vi "Configure Voltage Output.vi"(7 "Triggered Voltage (0 V)":dbl, 8 "error in (no error)":errorcluster, 9 "Immediate Voltage (0 V)":dbl, 10 "Transient Mode (0: Fixed)":i32(ring) items=["Fixed", "Step"], 11 "VISA resource name":refnum<visa-resource-name>) -> (0 "error out":errorcluster, 3 "VISA resource name out":refnum<visa-resource-name>)   [LabVIEW 2017, in "Keysight N8900 Series.lvlib"]
doc: "Configures the voltage transient mode and output voltage level."
uses:
  Keysight N8900 Series.lvlib
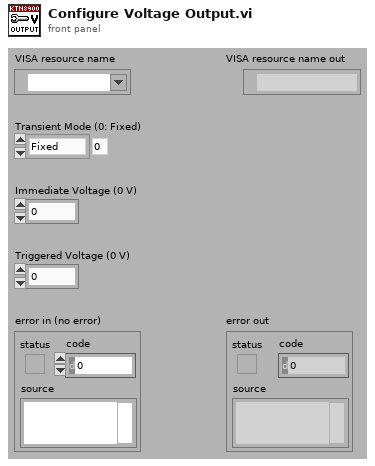
[diagram p1: front panel]
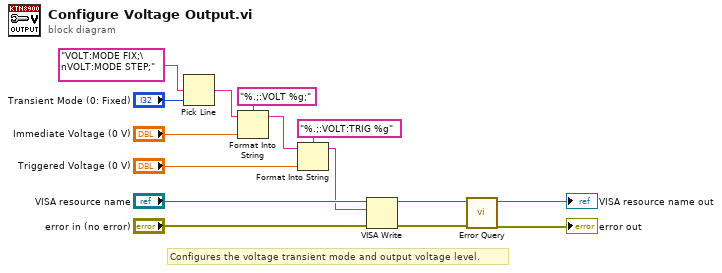
[diagram p0: block diagram]
diagram:
  # "Configures the voltage transient mode and output voltage level."
  n1 = Pick Line(multi-line string="VOLT:MODE FIX;\nVOLT:MODE STEP;", line index="Transient Mode (0: Fixed)") -> (output string=w6:string)  [unwired: 1 in]
  n2 = Format Into String(format string="%.;:VOLT %g;", initial string=w6, "Immediate Voltage (0 V)") -> (resulting string=w4:string)  [unwired: 1 in, 1 out]
  n3 = Format Into String(format string="%.;:VOLT:TRIG %g", initial string=w4, "Triggered Voltage (0 V)") -> (resulting string=w1:string)  [unwired: 1 in, 1 out]
  n4 = VISA Write(VISA resource name="VISA resource name", write buffer=w1, error in (no error)="error in (no error)") -> (VISA resource name out=w11:refnum<visa-resource-name>, error out=w10:errorcluster)  [unwired: 1 out]
  n5 = call "Error Query.vi"("error in (no error)"=w10, "VISA resource name"=w11) -> ("error out"=→"error out":errorcluster, "VISA resource name out"=→"VISA resource name out":refnum<visa-resource-name>)  [unwired: 6 in, 2 out]
